vi "Path Setup Callback Template.vi"(0 "RFCalAndFixtureCharact.Common.lvlib:Path.lvclass":refnum<class "Path.lvclass">, 5 "TSM Context":T1, 11 "error in":errorcluster) -> (15 "error out":errorcluster)   [LabVIEW 2023]
uses:
  Common/Base Classes/Path/Path.lvclass
  <vilib>/NI_TestStand_SemiconductorModule/NI_TestStand_Semiconductor_Module.lvlibp/PinMap/General/SemiconductorModuleContext.ctl
  <vilib>/NI_TestStand_SemiconductorModule/NI_TestStand_Semiconductor_Module.lvlibp
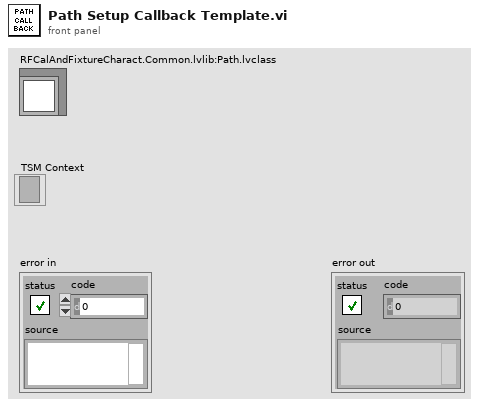
[diagram p1: front panel]
types:
  T1 = typedef "NI_TestStand_Semiconductor_Module.lvlibp/SemiconductorModuleContext.ctl" = refnum<k7>
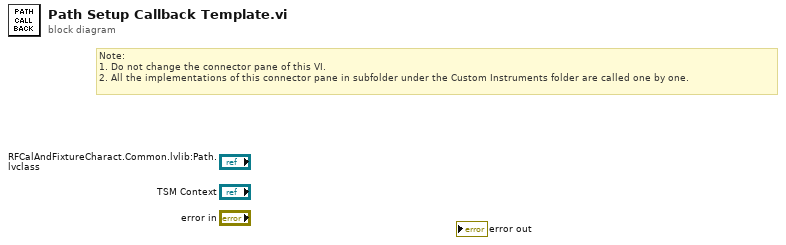
[diagram p0: block diagram]
diagram:
  # "Note: \n1. Do not change the connector pane of this VI.\n2. All the implementations of this connector pane in subfolder under the Custom Instruments folder are called one by one."
